vi "MTFileExistAddOne.vi"() -> ()   [LabVIEW 2012]
uses:
  Global1.vi
panel:
  in  "input string":string="2014/10/03"
  out "appended path":path
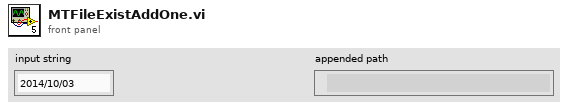
[diagram p1: front panel]
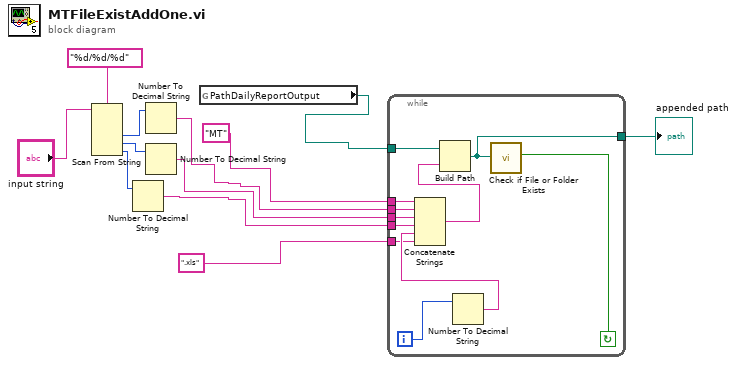
[diagram p0: block diagram]
diagram:
  n1 = Scan From String(format string="%d/%d/%d", input string="input string") -> (output 1=w11:i32, output 2=w10:i32, output 3=w9:i32)  [unwired: 5 in, 3 out]
  n2 = Number To Decimal String(number=w9) -> (decimal integer string=w2:string)  [unwired: 1 in]
  n3 = Number To Decimal String(number=w11) -> (decimal integer string=w4:string)  [unwired: 1 in]
  n4 = Number To Decimal String(number=w10) -> (decimal integer string=w3:string)  [unwired: 1 in]
  n5 = global read "Global1.vi" "PathDailyReportOutput"() -> (w7:path)
  n6 = while {
    tunnel: w7 -> [w23]
    tunnel: [w21] -> w6
    tunnel: "MT" ("string") -> [w19]
    tunnel: w4 -> [w18]
    tunnel: w3 -> [w17]
    tunnel: w2 -> [w16]
    tunnel: ".xls" ("string") -> [w14]
    i -> [w20]
    stop <- w22 continue-if-true
    n7 = Number To Decimal String(number=w20) -> (decimal integer string=w15:string)  [unwired: 1 in]
    n8 = Concatenate Strings(w19, w18, w17, w16, w15, w14) -> (w13:string)
    n9 = Build Path(base path=w23, name or relative path=w13) -> (appended path=w21:path)
    n10 = call <vilib>:"Check if File or Folder Exists.vi"("path"=w21) -> ("file or folder exists?"=w22:bool)  [unwired: 8 in, 2 out]
  }
  "appended path" <- w6
